vi "Acquire.vi"(6 "Integration Time":i32, 7 "MeasureControl":refnum<vi>, 8 "error in (no error)":errorcluster, 11 "Instruments in":refnum<class "Instruments.lvclass">) -> (0 "error out":errorcluster, 1 "20mA Spectra":cluster{"Wavelength":dbl[], "EL Spectrum":dbl[]}, 2 "Data Out":T1 {"50mA Data"."Current,mA" format="%_6g"; "50mA Data"."WL" format="%_6g"; "50mA Data"."Voltage" format="%_6g"; "50mA Data"."Power" format="%_6g"; "20mA Data"."Reverse" format="%#_3g"; "20mA Data"."Current,mA" format="%_6g"; "20mA Data"."Knee Current" format="%#_3g"; "20mA Data"."WL" format="%_6g"; "20mA Data"."Voltage" format="%_6g"; "20mA Data"."Power" format="%_5g"}, 3 "Instruments out":refnum<class "Instruments.lvclass">, 4 "50mA Spectra":cluster{"Wavelength":dbl[], "EL Spectrum":dbl[]}, 5 "remeasure?":bool)   [LabVIEW 2012, in "Instruments.lvclass"]
uses:
  Instruments.lvclass
  Controls/TestData.ctl
  Controls/MeasureControl.ctl
  Controls/TestArea.ctl
  Instruments.lvclass/Instruments.ctl
panel:
  out "Raw 2":dbl format="%0.2f"
  # "Current Result"
  # "Measure Control"
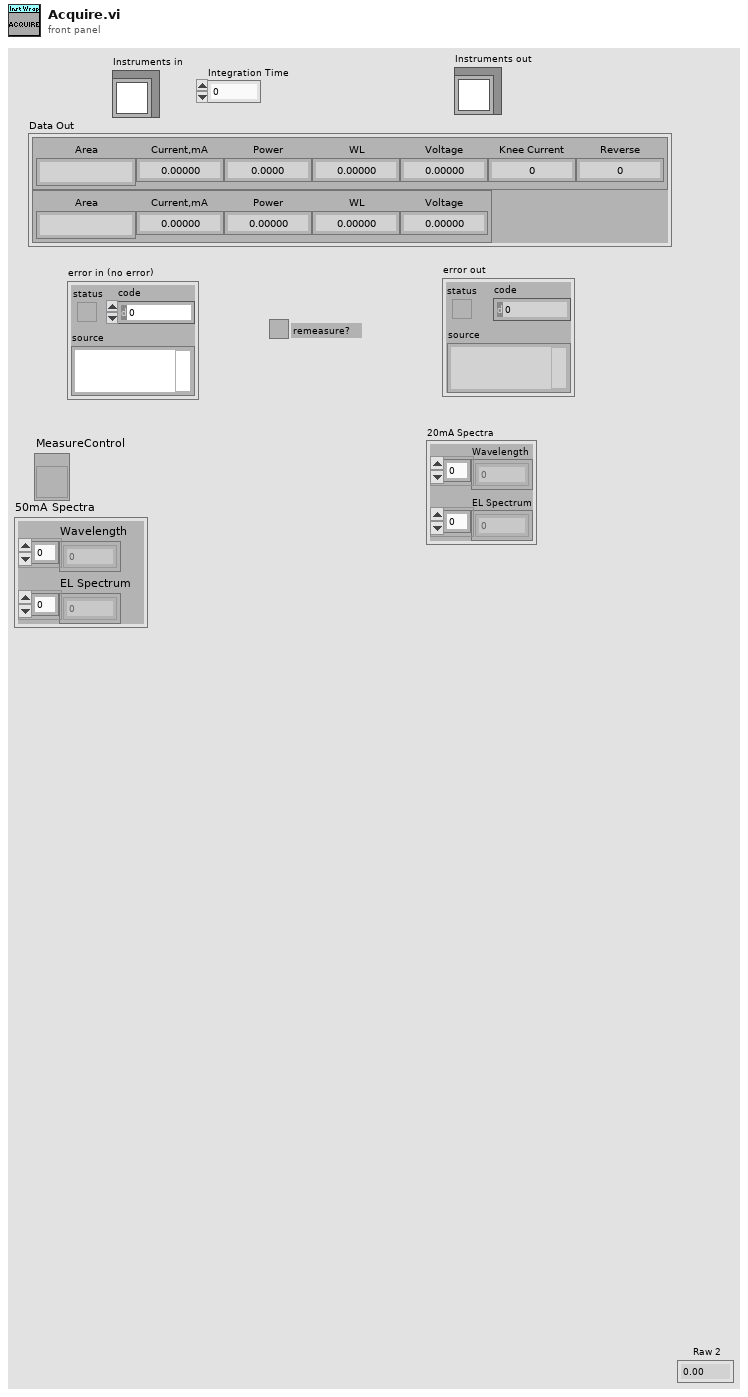
[diagram p1: front panel]
types:
  T1 = typedef "TestData.ctl" = cluster{"20mA Data":cluster{"Area":string, "Current,mA":dbl, "Power":dbl, "WL":dbl, "Voltage":dbl, "Knee Current":dbl, "Reverse":dbl}, "50mA Data":cluster{"Area":string, "Current,mA":dbl, "Power":dbl, "WL":dbl, "Voltage":dbl}}
  T2 = typedef "MeasureControl.ctl" = cluster{"Pass":bool, "Fail":bool, "Measure":bool, "Area":T3, "TestData":T1, "Graph":cluster{"Y":dbl[], "Y":dbl[]}[]}
  T3 = typedef "TestArea.ctl" = string
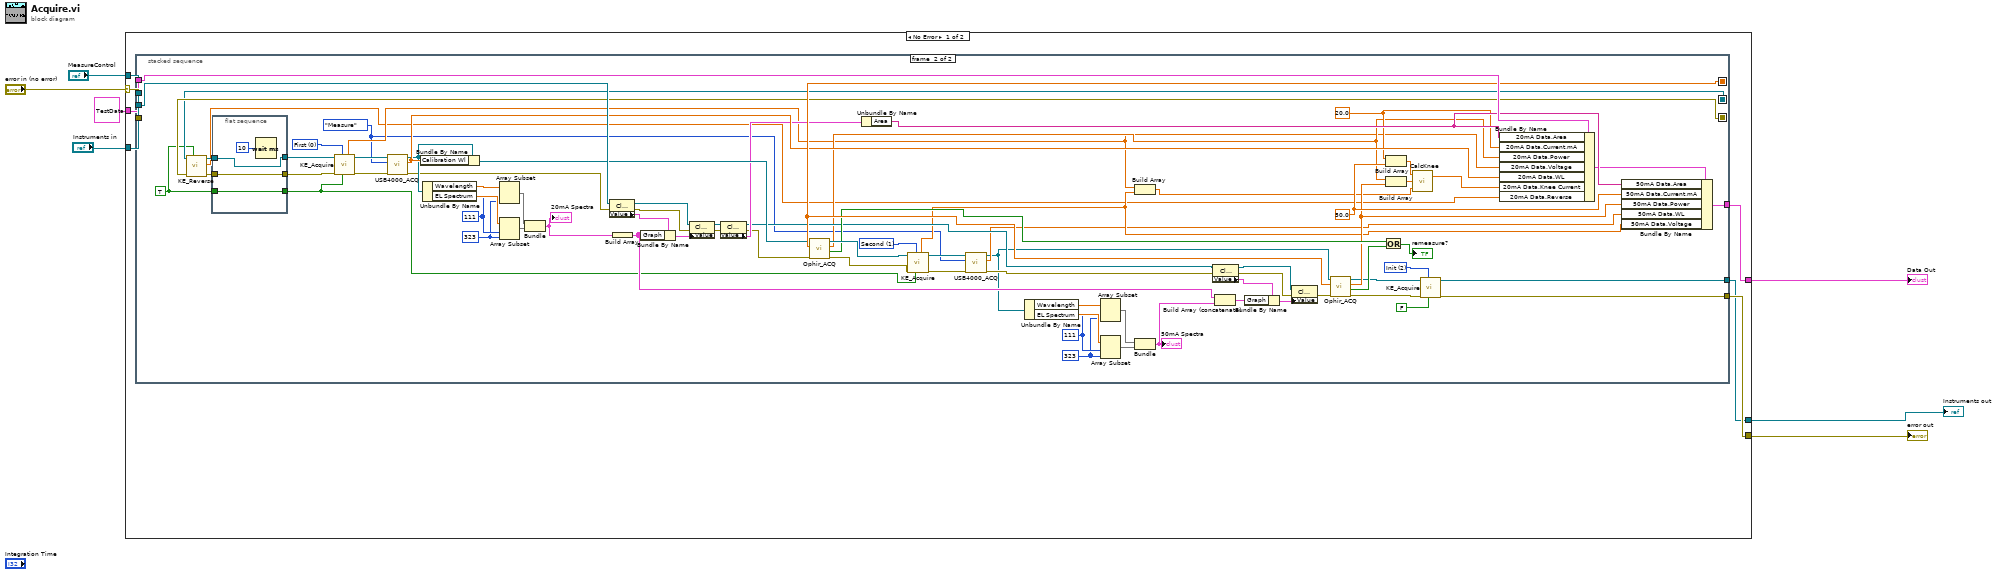
[diagram p0: block diagram]
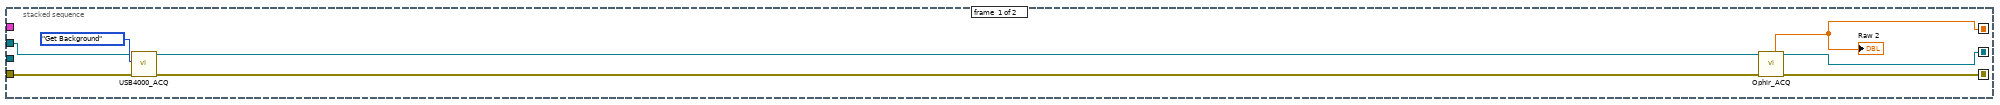
[diagram p2: hidden frame]
diagram:
  n1 = case shown="No Error" "error in (no error)" {
    selector: "error in (no error)" -> [w13 w108]
    tunnel: [w9 w108] -> w7
    tunnel: [w8 w107] -> w5
    tunnel: "Instruments in" -> [w14 w107]
    tunnel: [w11 _] -> w4
    tunnel: T1 {"20mA Data"={"Area"="", "Current,mA"=0.0, "Power"=0.0, "WL"=0.0, "Voltage"=0.0, "Knee Current"=0.0, "Reverse"=0.0}, "50mA Data"={"Area"="", "Current,mA"=0.0, "Power"=0.0, "WL"=0.0, "Voltage"=0.0}} ("TestData") -> [w12 _]
    tunnel: "MeasureControl" -> [w10 _]
    frame No Error {
      n2 = stacked-sequence {
        seq-local: [w22 _] -> [_ w100]
        seq-local: [w20 _] -> [_ w97]
        seq-local: [w21 _] -> [_ w98]
        tunnel: w14 -> [w16 _]
        tunnel: w13 -> [w15 _]
        tunnel: w12 -> [_ w102]
        tunnel: [_ w101] -> w11
        tunnel: w10 -> [_ w99]
        tunnel: [_ w95] -> w9
        tunnel: [_ w96] -> w8
        frame #0 {
          n3 = call-dynamic "USB4000_ACQ.vi"("error in (no error)"=w15, "Type"=enum16{"Get Background", "Measure"}."Get Background", "Instruments in"=w16) -> ("error out"=w17:errorcluster, "Instruments out"=w19:refnum<class "Instruments.lvclass">)  [unwired: 6 in, 1 out]
          n4 = call-dynamic "Ophir_ACQ.vi"("error in (no error)"=w17, "Instruments in"=w19) -> ("error out"=w21:errorcluster, "Instruments out"=w20:refnum<class "Instruments.lvclass">, "Back"=w22:dbl)  [unwired: 5 in, 2 out]
          "Raw 2" <- w22
        }
        frame #1 {
          w23 = enum16{"Get Background", "Measure", "Raw"}."Measure" ("Type")
          w36 = 323 ("length")
          w37 = 111 ("index")
          w42 = 323 ("length")
          w43 = 111 ("index")
          w47 = u16 2 items=["First", "Second", "Init"] ("Type")
          w27 = TRUE ("Boolean")
          w87 = u16 1 items=["First", "Second"] ("Type")
          w61 = 50.0 ("input variable")
          w60 = 20.0 ("input variable")
          w94 = u16 0 items=["First", "Second"] ("Type")
          n5 = call-dynamic "KE_Reverse.vi"("Boolean"=w27, "error in (no error)"=w98, "Instruments in"=w97) -> ("error out"=w30:errorcluster, "Current"=w26:dbl, "Instruments out"=w31:refnum<class "Instruments.lvclass">)  [unwired: 6 in]
          n6 = flat-sequence {
            tunnel: [w105] -> w32
            tunnel: w31 -> [w105]
            tunnel: w30 -> [w104]
            tunnel: [w104] -> w29
            tunnel: [w103] -> w28
            tunnel: w27 -> [w103]
            frame #0 {
              n7 = Wait (ms)(milliseconds to wait=u32 10) -> ()  [unwired: 1 out]
            }
          }
          n8 = call-dynamic "KE_Acquire.vi"("KeepOn?"=w28, "Type"=w94, "error in (no error)"=w29, "Instruments in"=w32) -> ("error out"=w92:errorcluster, "Instruments out"=w93:refnum<class "Instruments.lvclass">, "Voltage"=w57:dbl)  [unwired: 5 in]
          n9 = call-dynamic "USB4000_ACQ.vi"("error in (no error)"=w92, "Type"=w23, "Instruments in"=w93) -> ("error out"=w79:errorcluster, "Peak Wl"=w85:dbl, "Instruments out"=w84:refnum<class "Instruments.lvclass">)  [unwired: 6 in]
          n10 = Bundle By Name(cluster=w84, "Calibration Wl"=w85) -> (w91:refnum<class "Instruments.lvclass">)
          n11 = Unbundle By Name(w84) -> ("Wavelength"=w45:dbl[], "EL Spectrum"=w44:dbl[])
          n12 = Array Subset(array=w45, index=w43, length=w42) -> (w41:dbl[])
          n13 = Array Subset(array=w44, index=w43, length=w42) -> (w40:dbl[])
          n14 = Bundle(w41, w40) -> (w51:cluster{dbl[], dbl[]})  [unwired: 1 in]
          "20mA Spectra" <- w51
          n15 = property class="Clust (strict)"(reference=w99, error in=w79) -> (reference out=w81:refnum<vi>, error out=w80:errorcluster, "Value"=w83:T2)
          n16 = Build Array(w51) -> (w68:cluster{dbl[], dbl[]}[])
          n17 = Bundle By Name(cluster=w83, "Graph"=w68) -> (w82:T2)
          n18 = property class="Clust (strict)"(reference=w81, error in=w80, "Value"=w82) -> (reference out=w65:refnum<vi>, error out=w64:errorcluster)
          n19 = property class="Clust (strict)"(reference=w65, error in=w64) -> (reference out=w66:refnum<vi>, error out=w76:errorcluster, "Value"=w78:T2)
          n20 = call-dynamic "Ophir_ACQ.vi"("error in (no error)"=w76, "Background"=w100, "Instruments in"=w91) -> ("error out"=w86:errorcluster, "Remeasure?"=w75:bool, "Power,uW"=w59:dbl, "Instruments out"=w88:refnum<class "Instruments.lvclass">)  [unwired: 4 in, 1 out]
          n21 = Unbundle By Name(w78) -> ("Area"=w77:T3)
          n22 = call-dynamic "KE_Acquire.vi"("KeepOn?"=w28, "Type"=w87, "error in (no error)"=w86, "Instruments in"=w88) -> ("error out"=w90:errorcluster, "Instruments out"=w89:refnum<class "Instruments.lvclass">, "Voltage"=w56:dbl)  [unwired: 5 in]
          n23 = call-dynamic "USB4000_ACQ.vi"("error in (no error)"=w90, "Type"=w23, "Instruments in"=w89) -> ("error out"=w63:errorcluster, "Peak Wl"=w33:dbl, "Instruments out"=w24:refnum<class "Instruments.lvclass">)  [unwired: 6 in]
          n24 = Unbundle By Name(w24) -> ("Wavelength"=w39:dbl[], "EL Spectrum"=w38:dbl[])
          n25 = Array Subset(array=w39, index=w37, length=w36) -> (w35:dbl[])
          n26 = Array Subset(array=w38, index=w37, length=w36) -> (w34:dbl[])
          n27 = Build Array(w57, w56) -> (w53:dbl[])
          n28 = Bundle(w35, w34) -> (w46:cluster{dbl[], dbl[]})  [unwired: 1 in]
          "50mA Spectra" <- w46
          n29 = property class="Clust (strict)"(reference=w66, error in=w63) -> (reference out=w71:refnum<vi>, error out=w72:errorcluster, "Value"=w69:T2)
          n30 = Build Array (concatenate)(w68, w46) -> (w67:cluster{dbl[], dbl[]}[])
          n31 = Bundle By Name(cluster=w69, "Graph"=w67) -> (w70:T2)
          n32 = property class="Clust (strict)"(reference=w71, error in=w72, "Value"=w70) -> (error out=w62:errorcluster)  [unwired: 1 out]
          n33 = call-dynamic "Ophir_ACQ.vi"("error in (no error)"=w62, "Background"=w100, "Instruments in"=w24) -> ("error out"=w48:errorcluster, "Remeasure?"=w74:bool, "Power,uW"=w58:dbl, "Instruments out"=w49:refnum<class "Instruments.lvclass">)  [unwired: 4 in, 1 out]
          n34 = Or(x=w75, y=w74) -> (x .or. y?=→"remeasure?":bool)
          n35 = Build Array(w60, w61) -> (w55:dbl[])
          n36 = Build Array(w59, w58) -> (w54:dbl[])
          n37 = call "CalcKnee.vi"("Voltage"=w53, "Power"=w54, "Current"=w55) -> ("Knee Current"=w52:dbl)  [unwired: 1 out]
          n38 = call-dynamic "KE_Acquire.vi"("KeepOn?"=FALSE ("source"), "Type"=w47, "error in (no error)"=w48, "Instruments in"=w49) -> ("error out"=w95:errorcluster, "Instruments out"=w96:refnum<class "Instruments.lvclass">)  [unwired: 5 in, 1 out]
          n39 = Bundle By Name(cluster=w102, "20mA Data.Area"=w77, "20mA Data.Current,mA"=w60, "20mA Data.Power"=w59, "20mA Data.Voltage"=w57, "20mA Data.WL"=w85, "20mA Data.Knee Current"=w52, "20mA Data.Reverse"=w26) -> (w25:T1)
          n40 = Bundle By Name(cluster=w25, "50mA Data.Area"=w77, "50mA Data.Current,mA"=w61, "50mA Data.Power"=w58, "50mA Data.WL"=w33, "50mA Data.Voltage"=w56) -> (w101:T1)
        }
      }
    }
    frame Error {
    }
  }
  "error out" <- w7
  "Instruments out" <- w5
  "Data Out" <- w4
